vi "FPGA_I2C_Stop.vi"(10 "Wait Time":u32, 11 "IO Cluster":T1) -> (2 "Done?":bool)   [LabVIEW 2020]
doc: "Sends a stop bit to the slave device according to the I2C specifications."
uses:
  Controls/FPGA_I2C IO Cluster.ctl
  Controls/FPGA I2C_Stop State.ctl
  <vilib>/rvi/eio/common/nirviEmuTemplateMethod_errors.vi
  <vilib>/eio/EIOMethodNode/EIOMethodNode.xnode
  <vilib>/eio/EIONode/EIONode.xnode
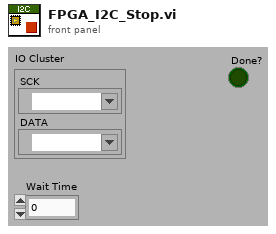
[diagram p1: front panel]
types:
  T1 = typedef "FPGA_I2C IO Cluster.ctl" = cluster{"SCK":refnum<k21>, "DATA":refnum<k21>}
  T2 = typedef "FPGA I2C_Stop State.ctl" = enum8{"Set DATA Low", "Wait 1", "Set CLK High", "Wait 2", "Set DATA High", "Wait 3", "Stop"}
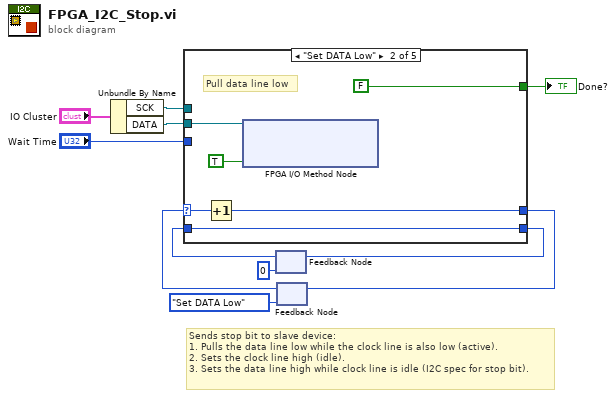
[diagram p0: block diagram]
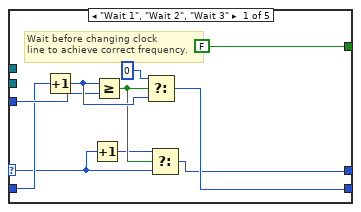
[diagram p2: hidden frame]
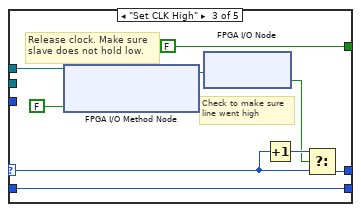
[diagram p3: hidden frame]
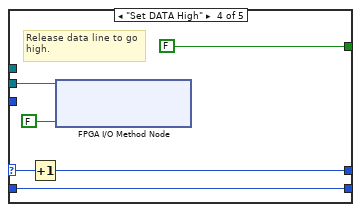
[diagram p4: hidden frame]
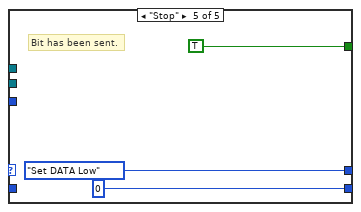
[diagram p5: hidden frame]
diagram:
  # "Sends stop bit to slave device:\n1. Pulls the data line low while the clock line is also low (active).\n2. Sets the clock line high (idle).\n3. Sets the data line high while clock line is idle (I2C spec for stop bit)."
  n1 = Unbundle By Name("IO Cluster") -> ("SCK"=w10:refnum<k21>, "DATA"=w9:refnum<k21>)
  n2 = feedback #1(u32 0 ("t")) -> (w4:u32)
  n3 = feedback #2(FPGA_I2C_Stop_State."Set DATA Low" ("State")) -> (w1:T2)
  n4 = case shown="\"Set DATA Low\"" w1 {
    selector: w1 -> [w14 w26 w30 w41 _]
    tunnel: [FALSE FALSE FALSE FALSE TRUE] -> w11
    tunnel: "Wait Time" -> [w19 _ _ _ _]
    tunnel: [w18 w24 w36 w39 u32 0 ("t")] -> w3
    tunnel: w4 -> [w17 w24 w36 w39 _]
    tunnel: [w13 w25 w28 w40 FPGA_I2C_Stop_State."Set DATA Low" ("State")] -> w6
    tunnel: w9 -> [_ w23 _ w38 _]
    tunnel: w10 -> [_ _ w29 _ _]
    frame "Wait 1", "Wait 2", "Wait 3" {
      # "Wait before changing clock\nline to achieve correct frequency."
      n5 = Increment(x=w17) -> (x+1=w20:u32)
      n6 = Increment(x=w14) -> (x+1=w15:T2)
      n7 = Greater Or Equal?(x=w20, y=w19) -> (x >= y?=w16:bool)
      n8 = Select(t=u32 0, s=w16, f=w20) -> (s? t:f=w18:u32)
      n9 = Select(t=w15, s=w16, f=w14) -> (s? t:f=w13:T2)
    }
    frame "Set DATA Low" {
      # "Pull data line low"
      n10 = Increment(x=w26) -> (x+1=w25:T2)
      n11 = xnode "FPGA I/O Method Node"("FPGA I/O In"=w23, "Enable"=TRUE) -> ()  [unwired: 1 out]
    }
    frame "Set CLK High" {
      # "Release clock. Make sure\nslave does not hold low."
      # "Check to make sure line went high"
      n12 = xnode "FPGA I/O Method Node"("FPGA I/O In"=w29, "Enable"=FALSE) -> ("FPGA I/O Out"=w34:refnum<k21>)
      n13 = xnode "FPGA I/O Node"("FPGA I/O In"=w34) -> ("I/O Item"=w31:bool)  [unwired: 1 out]
      n14 = Increment(x=w30) -> (x+1=w32:T2)
      n15 = Select(t=w32, s=w31, f=w30) -> (s? t:f=w28:T2)
    }
    frame "Set DATA High" {
      # "Release data line to go\nhigh."
      n16 = Increment(x=w41) -> (x+1=w40:T2)
      n17 = xnode "FPGA I/O Method Node"("FPGA I/O In"=w38, "Enable"=FALSE) -> ()  [unwired: 1 out]
    }
    frame "Stop" {
      # "Bit has been sent."
    }
  }
  "Done?" <- w11
  n18 = feedback-in #1(w3) -> ()
  n19 = feedback-in #2(w6) -> ()
